vi "TCP Listen.vi"(7 "net address":u32, 8 "error in (no error)":errorcluster, 9 "timeout ms (wait forever: -1)":i32=-1, 10 "port":u16) -> (0 "error out":errorcluster, 1 "remote port":u16, 2 "remote address":string, 3 "connection ID":refnum<k5>)   [LabVIEW 2011]
doc: "Creates a listener and waits for an accepted TCP network connection at the specified <B>port</B>."
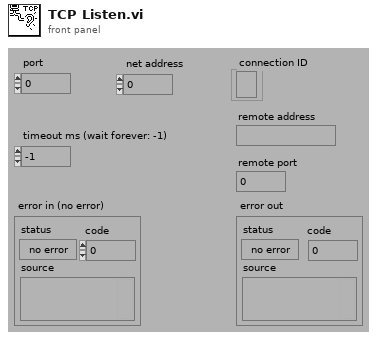
[diagram p1: front panel]
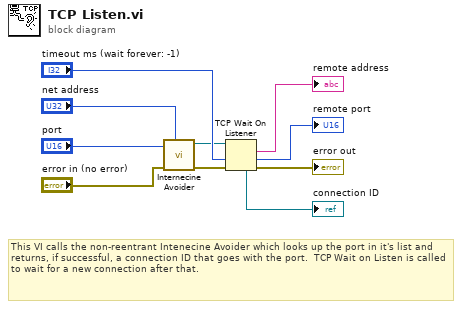
[diagram p0: block diagram]
diagram:
  # "This VI calls the non-reentrant Intenecine Avoider which looks up the port in it's list and returns, if successful, a connection ID that goes with the port.  TCP Wait on Listen is called to wait for a new connection after that."
  n1 = call "Internecine Avoider.vi"("net address"="net address", "error in (no error)"="error in (no error)", "port"="port") -> ("error out"=w3:errorcluster, "connection ID"=w4:refnum<k5>)  [unwired: 7 out]
  n2 = TCP Wait On Listener(8:w3, 9:"timeout ms (wait forever: -1)", 11:w4) -> (0:→"error out":errorcluster, 1:→"remote port":u16, 2:→"remote address":string, 4:→"connection ID":refnum<k5>)  [unwired: 2 out]
